vi "readHits.vi"(8 "Error In":errorcluster, 10 "#hits":i32, 11 "FGV_data":T2) -> (0 "Error Out":errorcluster, 1 "EOF":bool, 2 "hits":T1[](array[typedef]), 3 "FGV_data out":T2)   [LabVIEW 2018]
uses:
  FGV_data.ctl
  Config/config_data.ctl
  AE/hit_data.ctl
  AE/hit_raw_data.ctl
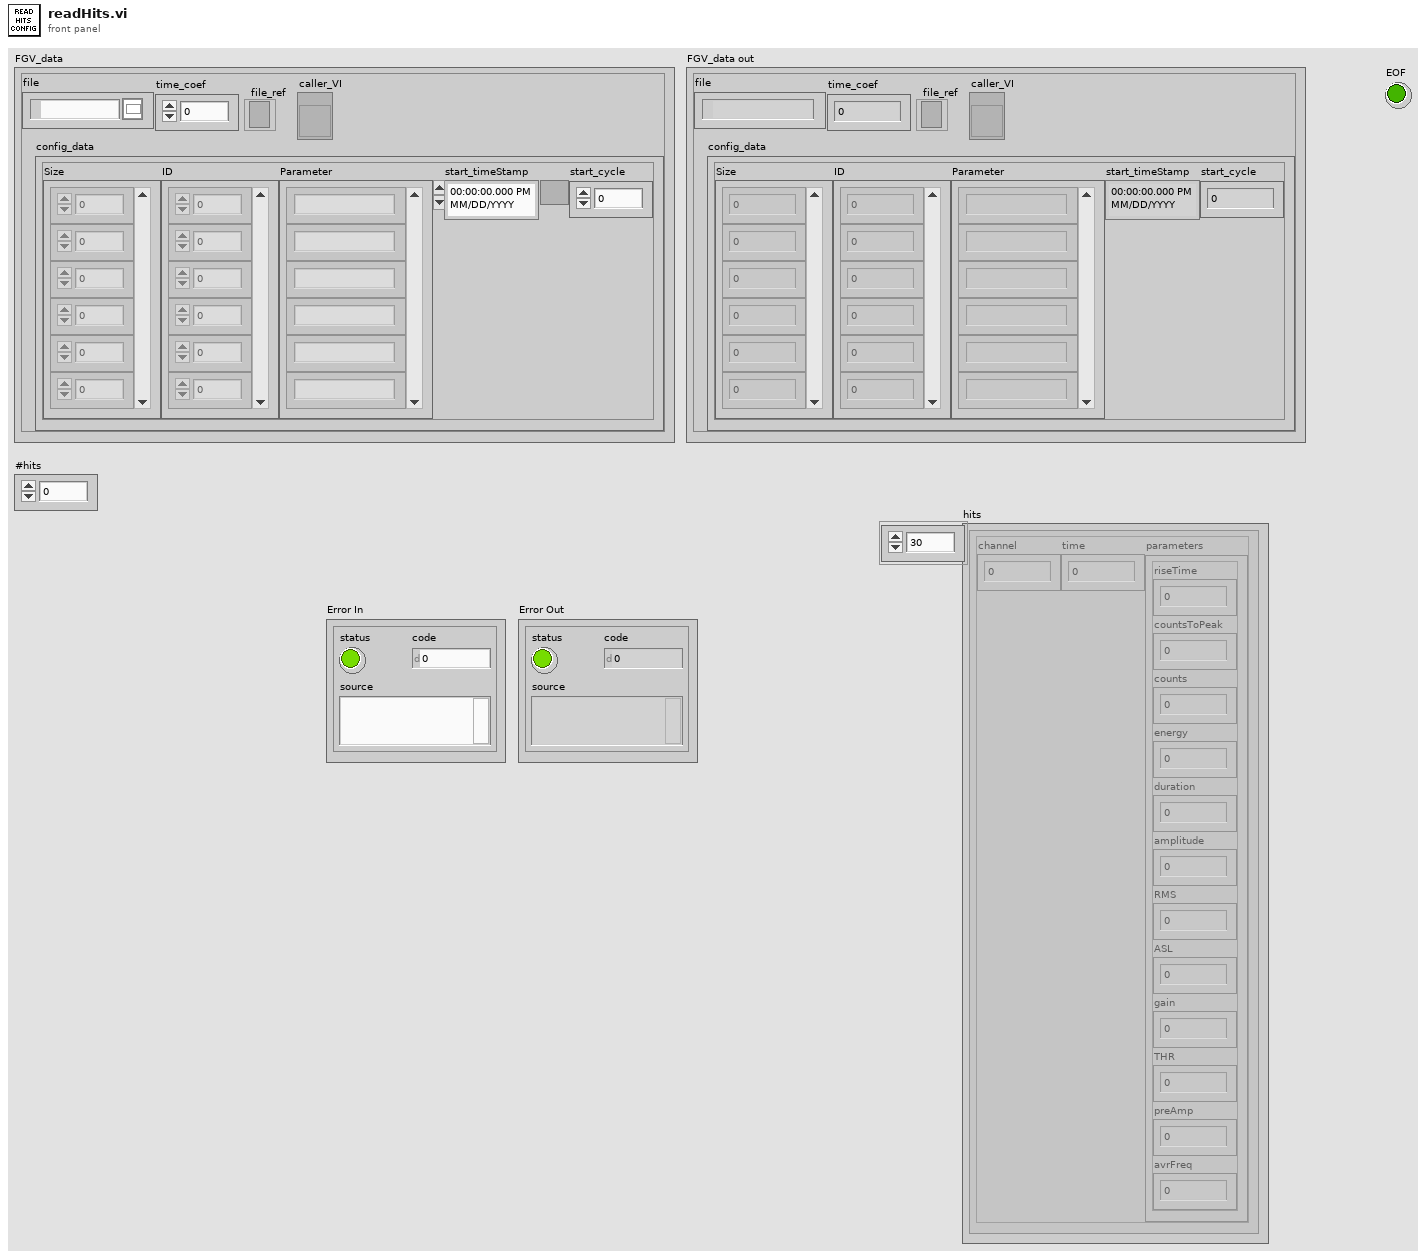
[diagram p1: front panel]
types:
  T1 = typedef "hit_data.ctl" = cluster{"channel":u8, "time":dbl, "parameters":cluster{"riseTime":u32, "countsToPeak":u32, "counts":u32, "energy":u32, "duration":u32, "amplitude":u32, "RMS":u32, "ASL":u32, "gain":u32, "THR":u32, "preAmp":u32, "avrFreq":u32}}
  T2 = typedef "FGV_data.ctl" = cluster{"file":path, "time_coef":dbl, "config_data":T3, "file_ref":refnum<file>, "caller_VI":refnum<vi>}
  T3 = typedef "config_data.ctl" = cluster{"Size":i32[], "ID":u8[], "Parameter":string[], "start_timeStamp":timestamp, "start_cycle":u64}
  T4 = typedef "hit_raw_data.ctl" = cluster{"channel":u8, "time":dbl, "data":u32[]}
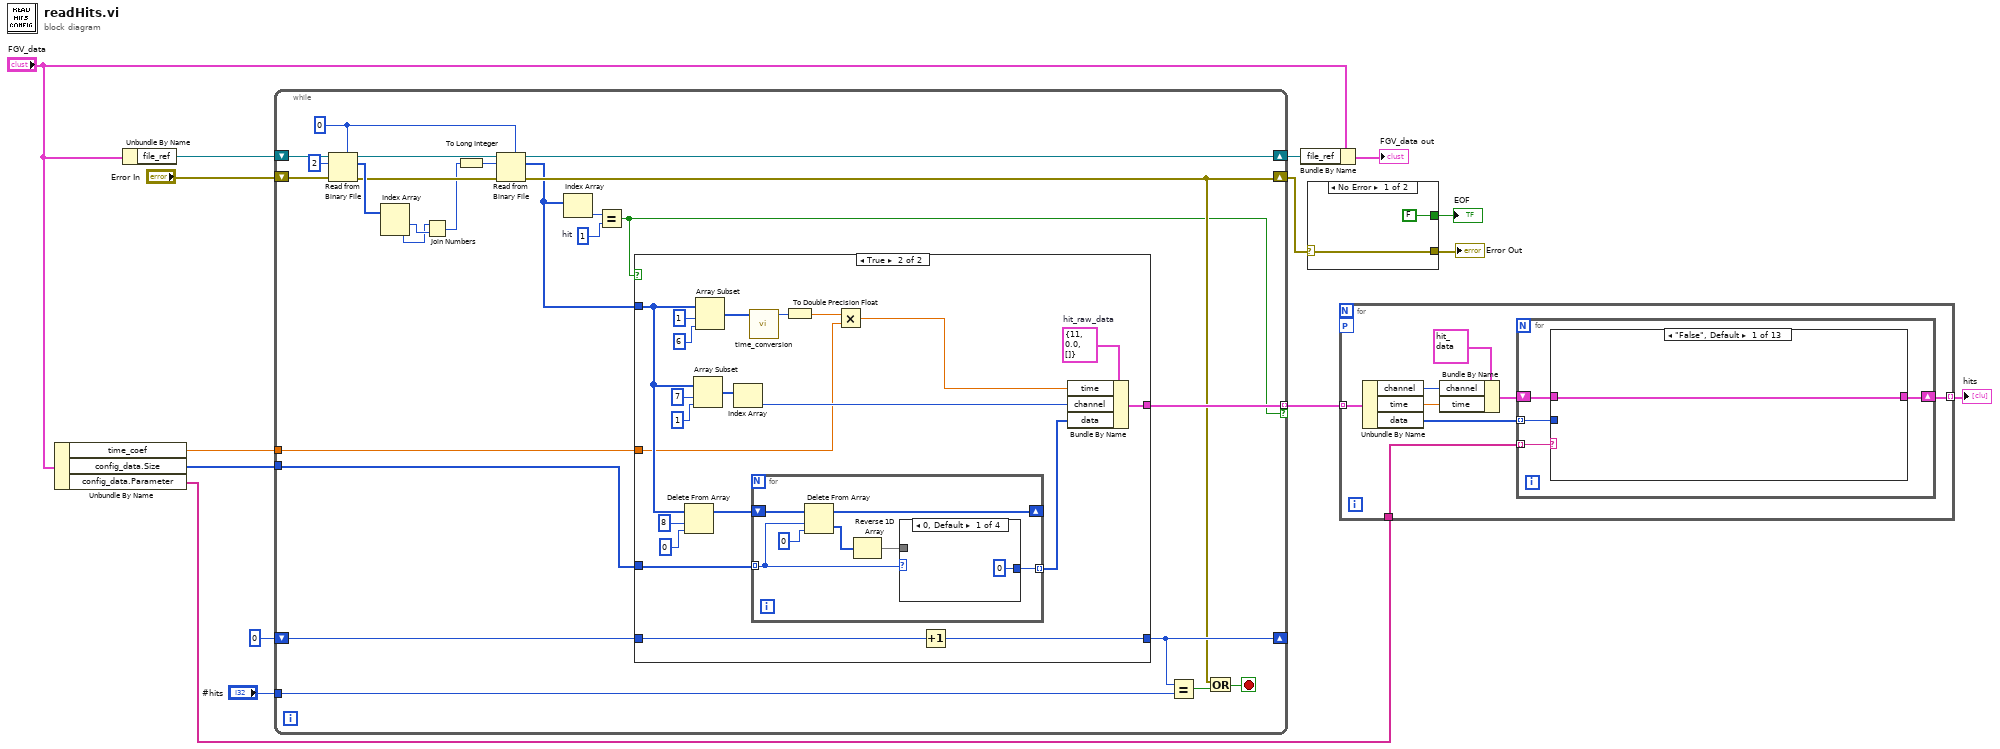
[diagram p0: block diagram]
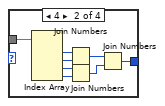
[diagram p3: hidden frame]
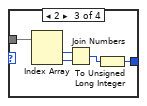
[diagram p4: hidden frame]
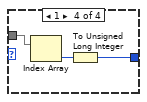
[diagram p5: hidden frame]
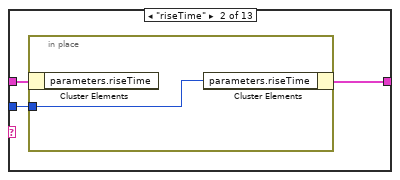
[diagram p6: hidden frame]
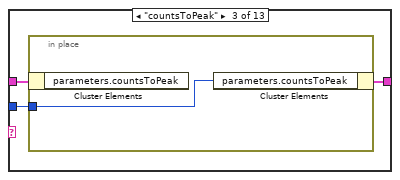
[diagram p7: hidden frame]
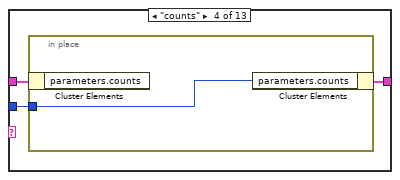
[diagram p8: hidden frame]
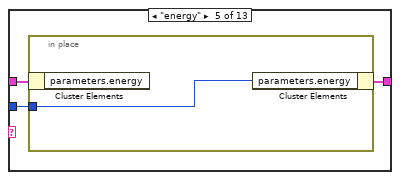
[diagram p9: hidden frame]
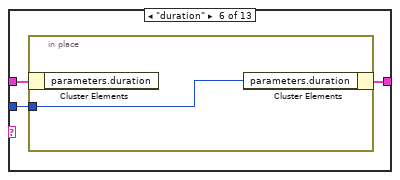
[diagram p10: hidden frame]
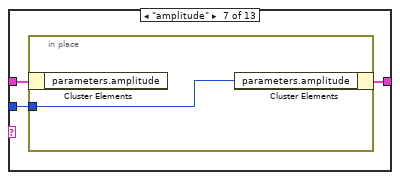
[diagram p11: hidden frame]
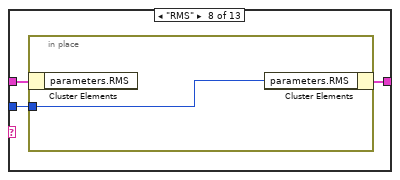
[diagram p12: hidden frame]
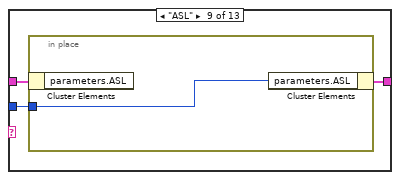
[diagram p13: hidden frame]
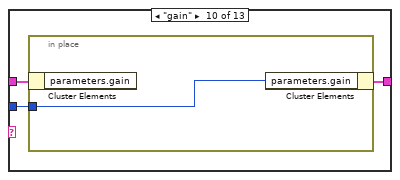
[diagram p14: hidden frame]
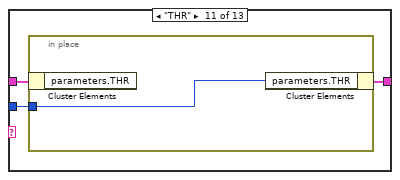
[diagram p15: hidden frame]
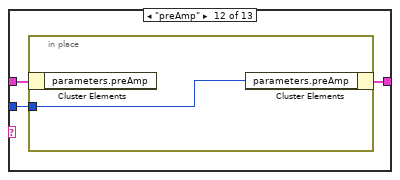
[diagram p16: hidden frame]
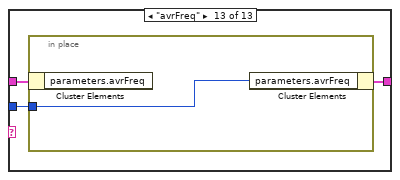
[diagram p17: hidden frame]
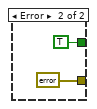
[diagram p18: hidden frame]
diagram:
  n1 = Unbundle By Name("FGV_data") -> ("time_coef"=w10:dbl, "config_data.Size"=w9:i32[], "config_data.Parameter"=w2:string[])
  n2 = Unbundle By Name("FGV_data") -> ("file_ref"=w15:refnum<file>)
  n3 = while {
    shift-right: [w18] -> w6
    shift-left: "Error In" -> [w32]
    tunnel: [w28] -> w3 mode=indexing if=w16
    shift-right: [w26] -> w13
    shift-left: w15 -> [w40]
    tunnel: w10 -> [w25]
    tunnel: w9 -> [w24]
    shift-right: [w22] -> _
    shift-left: 0 ("index") -> [w23]
    tunnel: "#hits" -> [w21]
    stop <- w19 stop-if-true
    w29 = u8 1  # hit
    w35 = u8 0
    n4 = Read from Binary File(5:w35, 8:w32, 10:2 ("count (1)"), 11:w40) -> (0:w36:errorcluster, 2:w38:u8[], 3:w37:refnum<file>)  [unwired: 2 in, 1 out]
    n5 = Index Array(array=w38) -> (element #1=w34:u8, element #2=w33:u8)  [unwired: 2 in]
    n6 = Join Numbers(hi=w33, lo=w34) -> ((hi.lo)=w31:u16)
    n7 = To Long Integer(number=w31) -> (32bit integer=w30:i32)
    n8 = Read from Binary File(5:w35, 8:w36, 10:w30, 11:w37) -> (0:w18:errorcluster, 2:w17:u8[], 3:w26:refnum<file>)  [unwired: 2 in, 1 out]
    n9 = Index Array(array=w17) -> (element=w27:u8)  [unwired: 1 in]
    n10 = Equal?(x=w27, y=w29) -> (x = y?=w16:bool)
    n11 = case shown="True" w16 {
      tunnel: w17 -> [_ w57]
      tunnel: [_ w51] -> w28
      tunnel: w24 -> [_ w50]
      tunnel: w25 -> [_ w42]
      tunnel: [w41 w48] -> w22
      tunnel: w23 -> [w41 w47]
      frame False {
      }
      frame True {
        w53 = T4 {"channel"=11, "time"=0.0, "data"=[]}  # hit_raw_data
        n12 = Delete From Array(array=w57, length=8 ("inicial"), index=0) -> (array with subset deleted=w54:u8[])  [unwired: 1 out]
        n13 = Array Subset(array=w57, index=7, length=1) -> (w58:u8[])
        n14 = Array Subset(array=w57, index=1, length=6) -> (w45:u8[])
        n15 = Index Array(array=w58) -> (element=w52:u8)  [unwired: 1 in]
        n16 = call "time_conversion.vi"("array_time"=w45) -> ("time_U64"=w43:u64)  [unwired: 10 in]
        n17 = for {
          shift-right: [w69] -> _
          shift-left: w54 -> [w67]
          tunnel: w50 -> [w64] mode=indexing
          tunnel: [w65] -> w49 mode=indexing
          n18 = Delete From Array(array=w67, length=w64, index=0) -> (deleted portion=w63:u8[], array with subset deleted=w69:u8[])
          n19 = Reverse 1D Array(array=w63) -> (reversed array=w66:u8[])
          n20 = case shown="0, Default" w64 {
            tunnel: w66 -> [_ w78 w83 w86]
            tunnel: [u32 0 w71 w79 w85] -> w65
            frame 0, Default {
            }
            frame 4 {
              n21 = Index Array(array=w78) -> (element #1=w74:u8, element #2=w75:u8, element #3=w76:u8, element #4=w77:u8)  [unwired: 4 in]
              n22 = Join Numbers(hi=w74, lo=w75) -> ((hi.lo)=w72:u16)
              n23 = Join Numbers(hi=w76, lo=w77) -> ((hi.lo)=w73:u16)
              n24 = Join Numbers(hi=w72, lo=w73) -> ((hi.lo)=w71:u32)
            }
            frame 2 {
              n25 = Index Array(array=w83) -> (element #1=w81:u8, element #2=w82:u8)  [unwired: 2 in]
              n26 = Join Numbers(hi=w81, lo=w82) -> ((hi.lo)=w80:u16)
              n27 = To Unsigned Long Integer(number=w80) -> (unsigned 32bit integer=w79:u32)
            }
            frame 1 {
              n28 = Index Array(array=w86) -> (element=w84:u8)  [unwired: 1 in]
              n29 = To Unsigned Long Integer(number=w84) -> (unsigned 32bit integer=w85:u32)
            }
          }
        }
        n30 = To Double Precision Float(number=w43) -> (double precision float=w46:dbl)
        n31 = Multiply(x=w46, y=w42) -> (x*y=w44:dbl)
        n32 = Increment(x=w47) -> (x+1=w48:i32)
        n33 = Bundle By Name(cluster=w53, "time"=w44, "channel"=w52, "data"=w49) -> (w51:T4)
      }
    }
    n34 = Equal?(x=w22, y=w21) -> (x = y?=w20:bool)
    n35 = Or(x=w18, y=w20) -> (x .or. y?=w19:bool)
  }
  n36 = Bundle By Name(cluster="FGV_data", "file_ref"=w13) -> (→"FGV_data out":T2)
  n37 = case shown="No Error" w6 {
    selector: w6 -> [w88 _]
    tunnel: [w88 errorcluster {"status"=FALSE, "code"=0, "source"=""} ("error IO")] -> w5
    tunnel: [FALSE ("EOF") TRUE ("EOF")] -> w4
    frame No Error {
    }
    frame Error {
    }
  }
  "Error Out" <- w5
  "EOF" <- w4
  n38 = for {
    tunnel: w3 -> [w98] mode=indexing
    tunnel: w2 -> [w93]
    tunnel: [w91] -> w1 mode=indexing
    workers-P: _ -> [_]
    n39 = Unbundle By Name(w98) -> ("channel"=w96:u8, "time"=w95:dbl, "data"=w92:u32[])
    n40 = Bundle By Name(cluster=T1 {"channel"=0, "time"=0.0, "parameters"={"riseTime"=0, "countsToPeak"=0, "counts"=0, "energy"=0, "duration"=0, "amplitude"=0, "RMS"=0, "ASL"=0, "gain"=0, "THR"=0, "preAmp"=0, "avrFreq"=0}} ("hit_data"), "channel"=w96, "time"=w95) -> (w94:T1)
    n41 = for {
      shift-right: [w99] -> w91
      shift-left: w94 -> [w102]
      tunnel: w93 -> [w101] mode=indexing
      tunnel: w92 -> [w100] mode=indexing
      n42 = case shown="\"False\", Default" w101 {
        tunnel: w102 -> [w103 w106 w110 w114 w118 w122 w126 w130 w134 w138 w142 w146 w150]
        tunnel: w100 -> [_ w105 w109 w113 w117 w121 w125 w129 w133 w137 w141 w145 w149]
        tunnel: [w103 w104 w108 w112 w116 w120 w124 w128 w132 w136 w140 w144 w148] -> w99
        frame "False", Default {
        }
        frame "riseTime" {
          n43 = in-place {
            in-place-border: w105 -> [w107]
            n44 = in-place-cluster #1(w106) -> ()  [unwired: 1 out]
            n45 = in-place-cluster #1("parameters.riseTime"=w107) -> (w104:T1)
          }
        }
        frame "countsToPeak" {
          n46 = in-place {
            in-place-border: w109 -> [w111]
            n47 = in-place-cluster #2(w110) -> ()  [unwired: 1 out]
            n48 = in-place-cluster #2("parameters.countsToPeak"=w111) -> (w108:T1)
          }
        }
        frame "counts" {
          n49 = in-place {
            in-place-border: w113 -> [w115]
            n50 = in-place-cluster #3(w114) -> ()  [unwired: 1 out]
            n51 = in-place-cluster #3("parameters.counts"=w115) -> (w112:T1)
          }
        }
        frame "energy" {
          n52 = in-place {
            in-place-border: w117 -> [w119]
            n53 = in-place-cluster #4(w118) -> ()  [unwired: 1 out]
            n54 = in-place-cluster #4("parameters.energy"=w119) -> (w116:T1)
          }
        }
        frame "duration" {
          n55 = in-place {
            in-place-border: w121 -> [w123]
            n56 = in-place-cluster #5(w122) -> ()  [unwired: 1 out]
            n57 = in-place-cluster #5("parameters.duration"=w123) -> (w120:T1)
          }
        }
        frame "amplitude" {
          n58 = in-place {
            in-place-border: w125 -> [w127]
            n59 = in-place-cluster #6(w126) -> ()  [unwired: 1 out]
            n60 = in-place-cluster #6("parameters.amplitude"=w127) -> (w124:T1)
          }
        }
        frame "RMS" {
          n61 = in-place {
            in-place-border: w129 -> [w131]
            n62 = in-place-cluster #7(w130) -> ()  [unwired: 1 out]
            n63 = in-place-cluster #7("parameters.RMS"=w131) -> (w128:T1)
          }
        }
        frame "ASL" {
          n64 = in-place {
            in-place-border: w133 -> [w135]
            n65 = in-place-cluster #8(w134) -> ()  [unwired: 1 out]
            n66 = in-place-cluster #8("parameters.ASL"=w135) -> (w132:T1)
          }
        }
        frame "gain" {
          n67 = in-place {
            in-place-border: w137 -> [w139]
            n68 = in-place-cluster #9(w138) -> ()  [unwired: 1 out]
            n69 = in-place-cluster #9("parameters.gain"=w139) -> (w136:T1)
          }
        }
        frame "THR" {
          n70 = in-place {
            in-place-border: w141 -> [w143]
            n71 = in-place-cluster #10(w142) -> ()  [unwired: 1 out]
            n72 = in-place-cluster #10("parameters.THR"=w143) -> (w140:T1)
          }
        }
        frame "preAmp" {
          n73 = in-place {
            in-place-border: w145 -> [w147]
            n74 = in-place-cluster #11(w146) -> ()  [unwired: 1 out]
            n75 = in-place-cluster #11("parameters.preAmp"=w147) -> (w144:T1)
          }
        }
        frame "avrFreq" {
          n76 = in-place {
            in-place-border: w149 -> [w151]
            n77 = in-place-cluster #12(w150) -> ()  [unwired: 1 out]
            n78 = in-place-cluster #12("parameters.avrFreq"=w151) -> (w148:T1)
          }
        }
      }
    }
  }
  "hits" <- w1
